vi "Sprinkler.vi"() -> ()   [LabVIEW 2024]
uses:
  Controls/Data Cluster.ctl
  <vilib>/Utility/error.llb/Error Cluster From Error Code.vi
  <vilib>/ErrorRing/Error Ring.xnode
panel:
  in  "Error In":errorcluster
  in  "Zone Setup Array":cluster{"Zone Selector":string, "Timing":dbl}[](array[cluster])
  out "Controller Status":string
  out "Zone Indicators":T1
  in  "Water Pressure Sensor (%)":u32(slide) scale=0.0..100.0
  in  "Rain Sensor":bool
  in  "Run Selector":bool
  in  "Setup":bool
  in  "Start":bool
  in  "stop":bool
  # "Controls"
  # "Simulation Controls"
  # "Rain"
  # "No Rain"
  # "Continuous"
  # "Single"
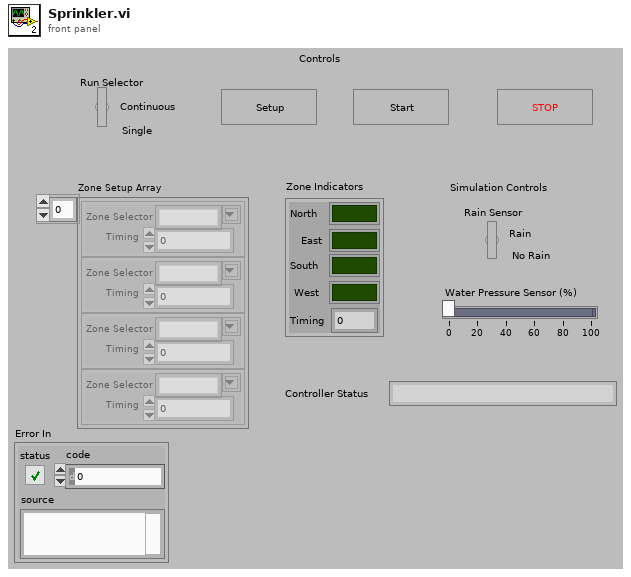
[diagram p1: front panel]
types:
  T1 = cluster{"North":bool, "East":bool, "South":bool, "West":bool, "Timing":u32}
  T2 = enum16{"Create", "Enqueue", "Dequeue", "Enstack", "Flush", "Release"}
  T3 = enum8{"Enabled", "Disabled", "Disabled and Grayed Out"}
  T4 = typedef "Data Cluster.ctl" = cluster{"Zone Setup Array Actual":cluster{"Zone Selector":string, "Timing":dbl}[], "Zone Setup Array Current":cluster{"Zone Selector":string, "Timing":dbl}[], "Zone Indicators":cluster{"North":bool, "East":bool, "South":bool, "West":bool, "Timing":u32}, "Controller Status":string, "Water Pressure Sensor (%)":u32, "Rain Sensor":bool, "Current Zone Active?":bool, "Time Elapsed?":bool, "QueueRefOut":refnum<queue>}
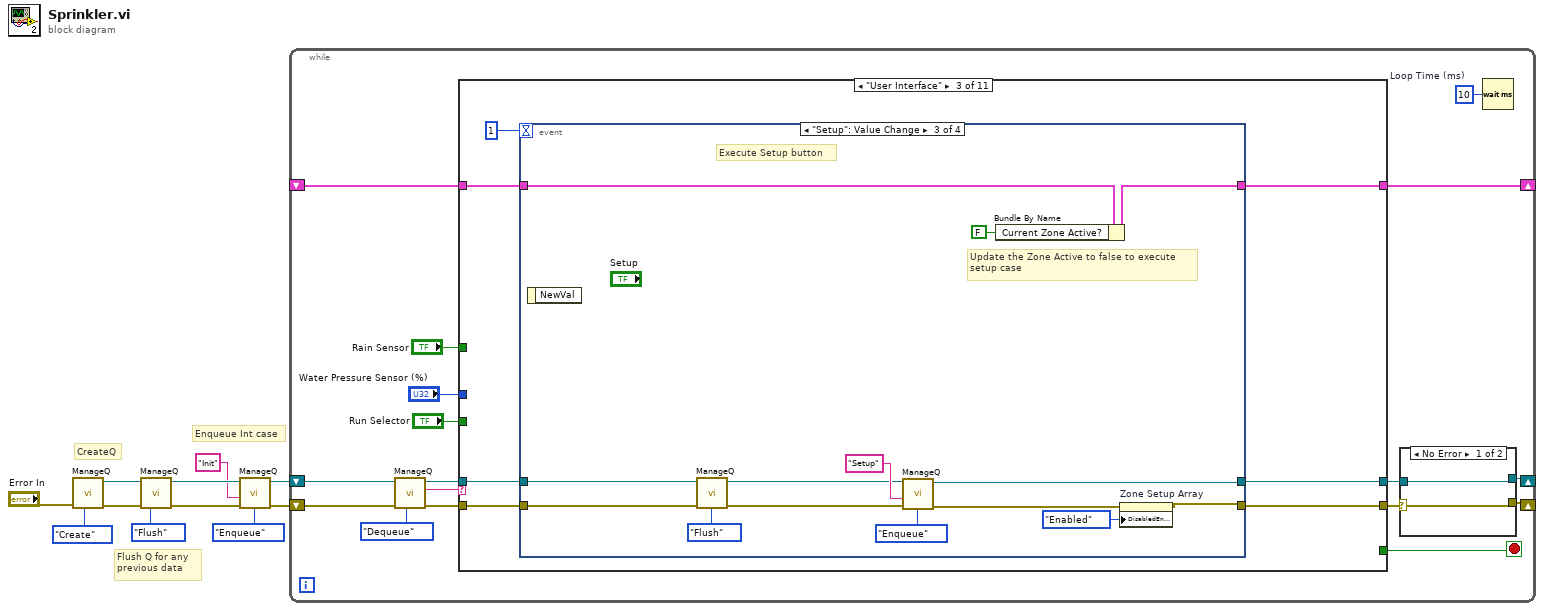
[diagram p0: block diagram]
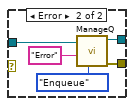
[diagram p2: hidden frame]
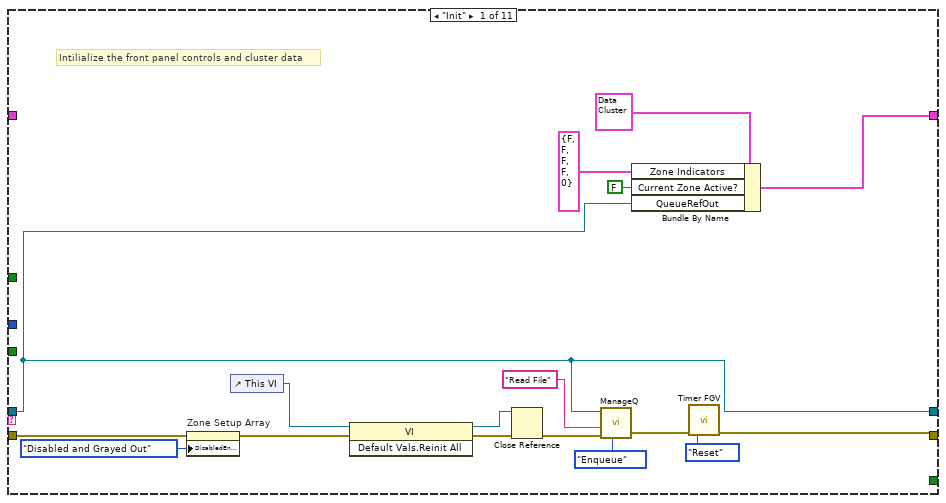
[diagram p3: hidden frame]
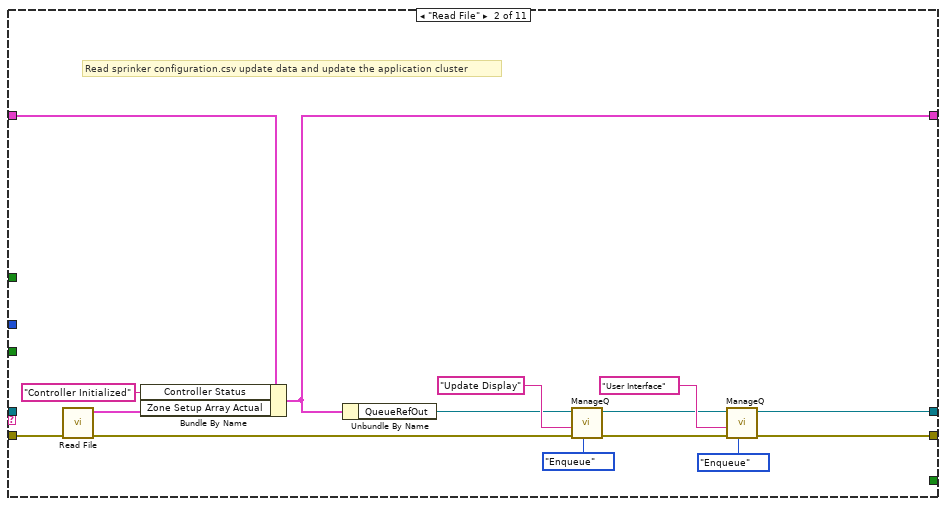
[diagram p4: hidden frame]
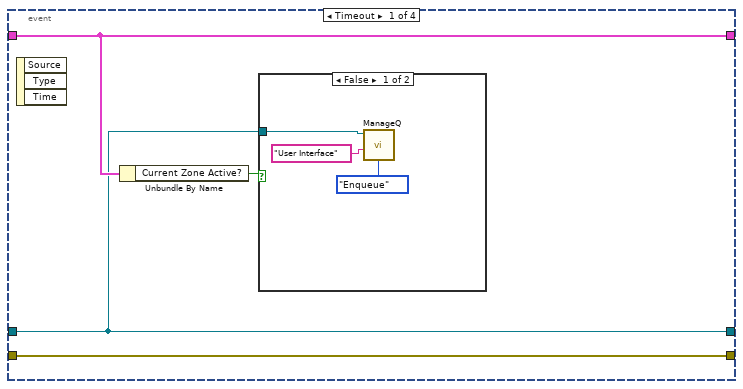
[diagram p5: hidden frame]
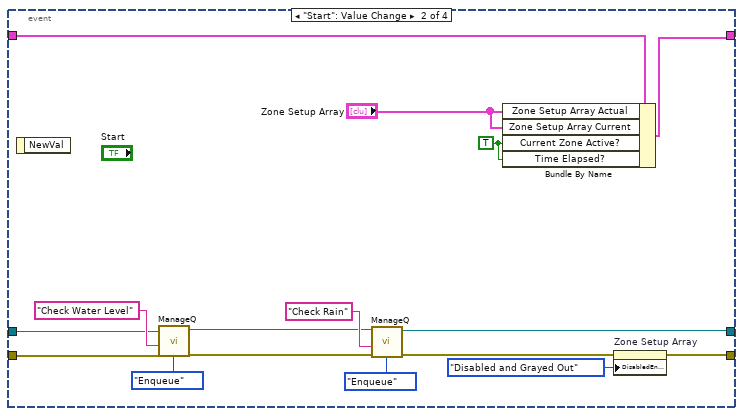
[diagram p7: hidden frame]
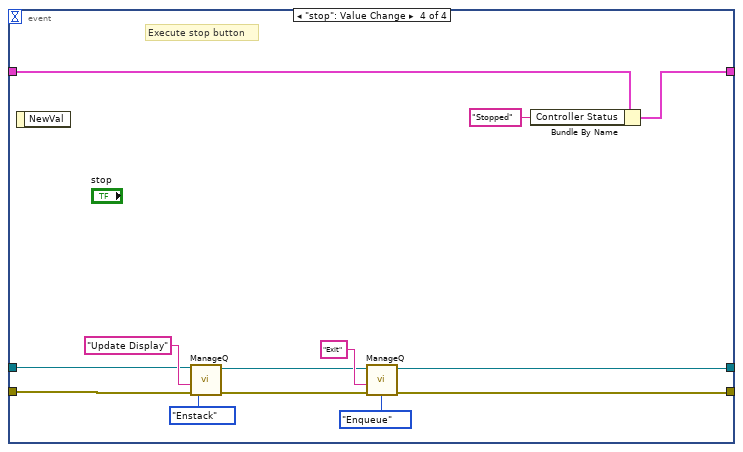
[diagram p8: hidden frame]
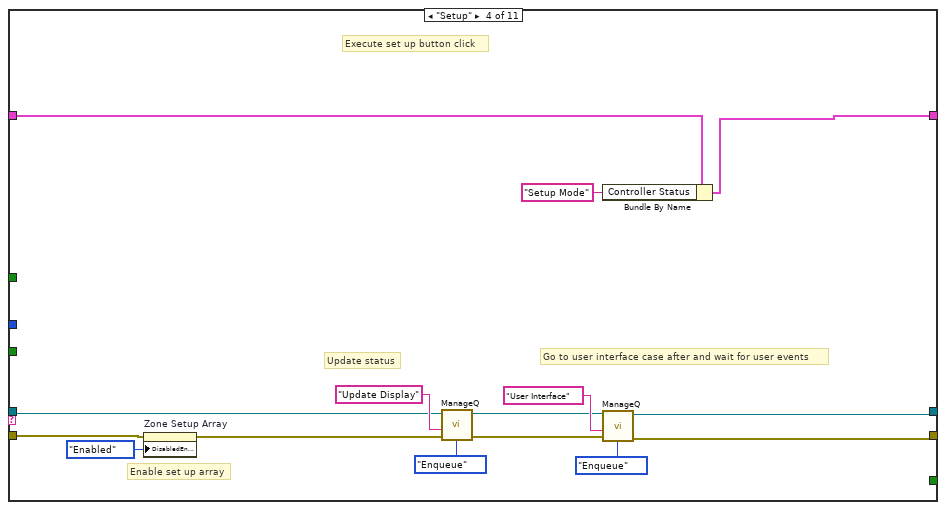
[diagram p9: hidden frame]
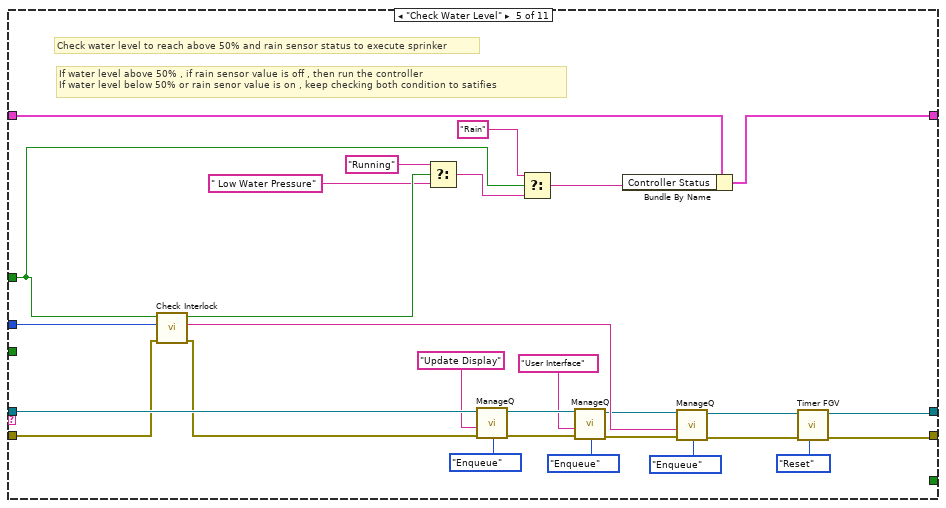
[diagram p10: hidden frame]
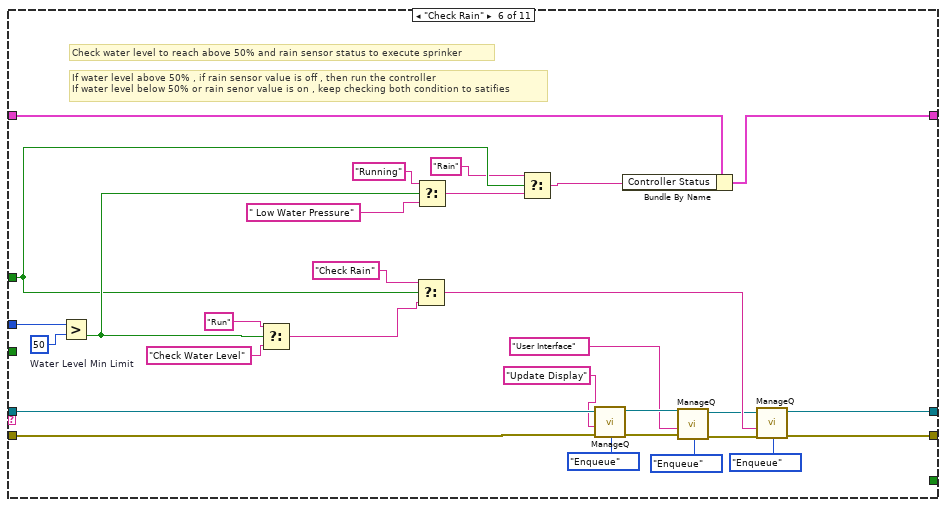
[diagram p11: hidden frame]
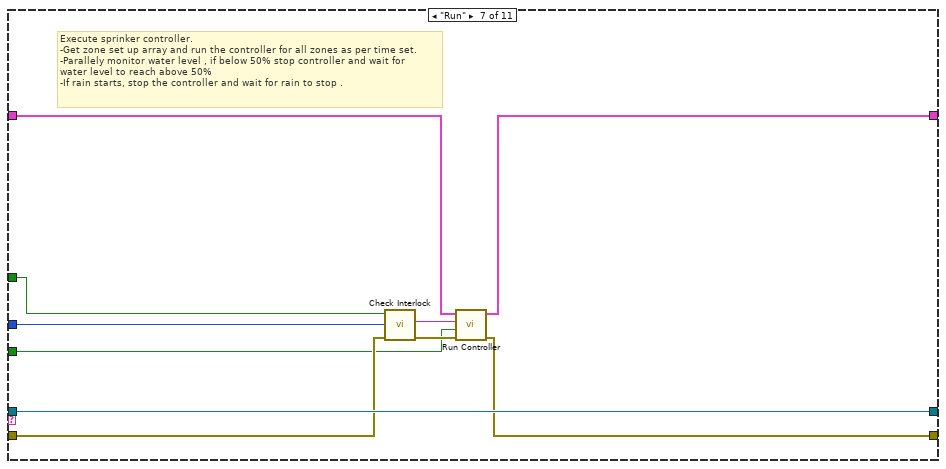
[diagram p12: hidden frame]
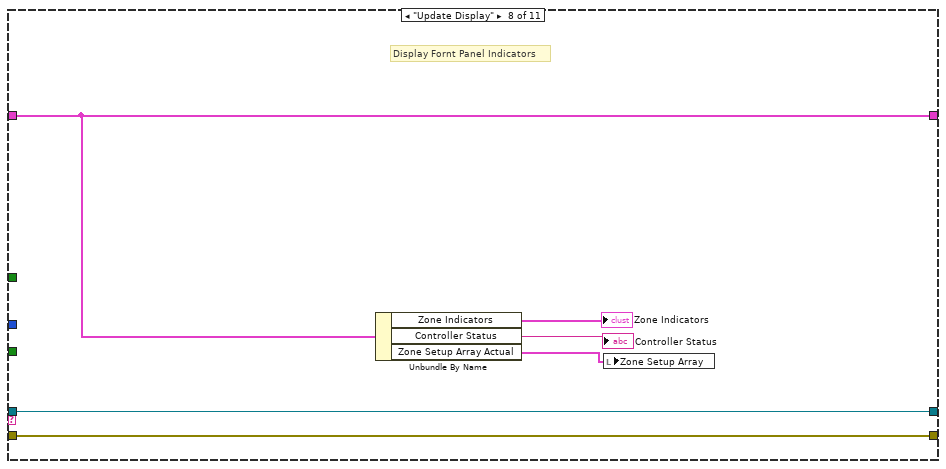
[diagram p13: hidden frame]
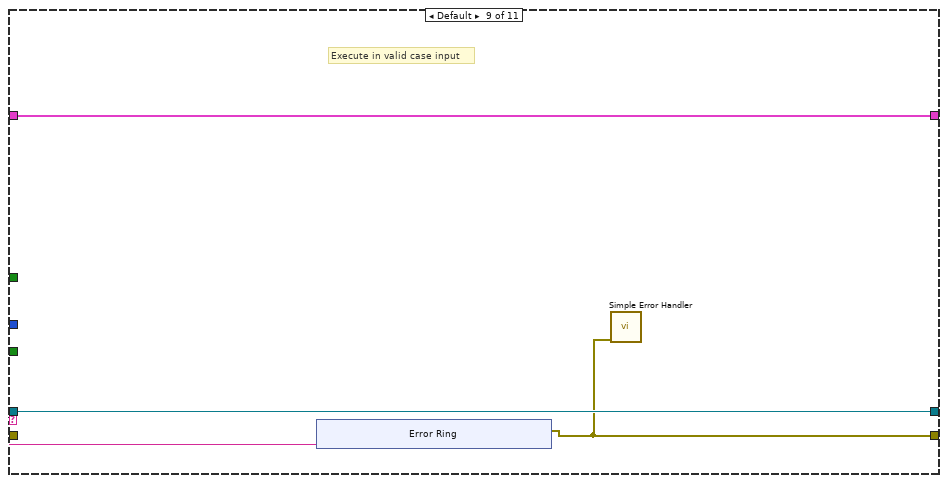
[diagram p14: hidden frame]
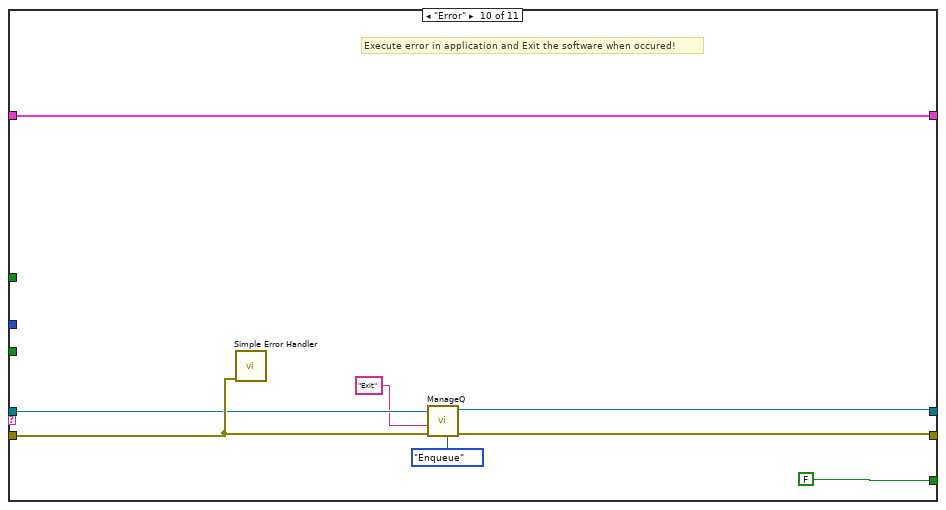
[diagram p15: hidden frame]
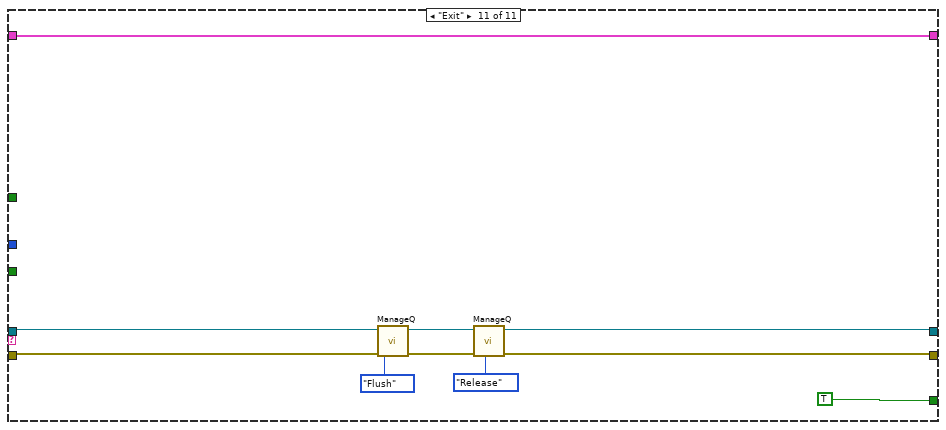
[diagram p16: hidden frame]
diagram:
  # "Enqueue Int case"
  # "Flush Q for any \nprevious data"
  # "CreateQ"
  n1 = call "ManageQ.vi"("QStateIn"=T2."Create", "Error In"="Error In") -> ("Error Out"=w9:errorcluster, "QueueRefOut"=w3:refnum<queue>)  [unwired: 7 in, 1 out]
  n2 = call "ManageQ.vi"("QStateIn"=T2."Flush", "Error In"=w9, "QueueRefIn"=w3) -> ("Error Out"=w8:errorcluster, "QueueRefOut"=w4:refnum<queue>)  [unwired: 6 in, 1 out]
  n3 = call "ManageQ.vi"("QStateIn"=T2."Enqueue", "Error In"=w8, "State In"="Init", "QueueRefIn"=w4) -> ("Error Out"=w7:errorcluster, "QueueRefOut"=w1:refnum<queue>)  [unwired: 5 in, 1 out]
  n4 = while {
    shift-right: [w19] -> _
    shift-left: w7 -> [w28]
    shift-right: [w21] -> _
    shift-left: _ -> [w22]
    shift-right: [w17] -> _
    shift-left: w1 -> [w26]
    stop <- w16 stop-if-true
    w15 = u32 10  # Loop Time (ms)
    n5 = call "ManageQ.vi"("QStateIn"=T2."Dequeue", "Error In"=w28, "QueueRefIn"=w26) -> ("Error Out"=w27:errorcluster, "State Out"=w24:string, "QueueRefOut"=w23:refnum<queue>)  [unwired: 6 in]
    n6 = case shown="\"User Interface\"" w24 {
      selector: w24 -> [_ _ _ _ _ _ _ _ w212 _ _]
      tunnel: w27 -> [w43 w67 w71 w138 w156 w192 w198 w210 _ w226 w236]
      tunnel: [w39 w55 w70 w133 w139 w191 w203 w210 w211 w223 w232] -> w20
      tunnel: w23 -> [w36 _ w72 w126 w164 w190 w204 w206 w213 w225 w237]
      tunnel: w22 -> [_ w66 w74 w131 w163 w186 w202 w209 w214 w229 w239]
      tunnel: [w45 w54 w73 w130 w157 w180 w201 w209 w214 w229 w239] -> w21
      tunnel: [w36 w58 w69 w134 w154 w189 w204 w206 w213 w224 w231] -> w18
      tunnel: [_ _ _ _ _ _ _ _ _ FALSE TRUE] -> w16
      tunnel: "Water Pressure Sensor (%)" -> [_ _ _ _ w165 w194 w199 _ _ _ _]
      tunnel: "Rain Sensor" -> [_ _ _ _ w159 w182 w200 _ _ _ _]
      tunnel: "Run Selector" -> [_ _ _ _ _ _ w195 _ _ _ _]
      frame "Init" {
        # "Intilialize the front panel controls and cluster data"
        n7 = property on="Zone Setup Array" class="Arr (strict)"(error in=w43, "DisabledEnum"=T3."Disabled and Grayed Out" ("Disabled")) -> (error out=w42:errorcluster)  [unwired: 1 in, 1 out]
        n8 = control-ref of="This VI"() -> (w52:refnum<vi>)
        n9 = invoke class="VI" method="Default Vals.Reinit All"(reference=w52, error in=w42) -> (reference out=w50:refnum<vi>, error out=w51:errorcluster)  [unwired: 1 in, 1 out]
        n10 = Close Reference(reference=w50, error in (no error)=w51) -> (error out=w49:errorcluster)
        n11 = call "ManageQ.vi"("QStateIn"=T2."Enqueue", "Error In"=w49, "State In"="Read File", "QueueRefIn"=w36) -> ("Error Out"=w40:errorcluster)  [unwired: 5 in, 2 out]
        n12 = Bundle By Name(cluster=T4 {"Zone Setup Array Actual"=[], "Zone Setup Array Current"=[], "Zone Indicators"={"North"=FALSE, "East"=FALSE, "South"=FALSE, "West"=FALSE, "Timing"=0}, "Controller Status"="", "Water Pressure Sensor (%)"=0, "Rain Sensor"=FALSE, "Current Zone Active?"=FALSE, "Time Elapsed?"=FALSE, "QueueRefOut"=refnum}, "Zone Indicators"=T1 {"North"=FALSE, "East"=FALSE, "South"=FALSE, "West"=FALSE, "Timing"=0}, "Current Zone Active?"=FALSE, "QueueRefOut"=w36) -> (w45:T4)
        n13 = call "Timer FGV.vi"("Error In"=w40, "Timer state"=enum16{"Reset", "Read", "Pause"}."Reset") -> ("Error Out"=w39:errorcluster)  [unwired: 7 in, 2 out]
      }
      frame "Read File" {
        # "Read sprinker configuration.csv update data and update the application cluster"
        n14 = call "Read File.vi"("Error In"=w67) -> ("Error Out"=w64:errorcluster, "Zone Set Up"=w65:cluster{"Zone Selector":string, "Timing":dbl}[])  [unwired: 9 in]
        n15 = Bundle By Name(cluster=w66, "Controller Status"="Controller Initialized", "Zone Setup Array Actual"=w65) -> (w54:T4)
        n16 = Unbundle By Name(w54) -> ("QueueRefOut"=w53:refnum<queue>)
        n17 = call "ManageQ.vi"("QStateIn"=T2."Enqueue", "Error In"=w64, "State In"="Update Display", "QueueRefIn"=w53) -> ("Error Out"=w56:errorcluster, "QueueRefOut"=w59:refnum<queue>)  [unwired: 5 in, 1 out]
        n18 = call "ManageQ.vi"("QStateIn"=T2."Enqueue", "Error In"=w56, "State In"="User Interface", "QueueRefIn"=w59) -> ("Error Out"=w55:errorcluster, "QueueRefOut"=w58:refnum<queue>)  [unwired: 5 in, 1 out]
      }
      frame "User Interface" {
        n19 = event shown="[2] \"Setup\": Value Change" {
          selector: _ -> [_ _ _ _]
          dyn-events: _ -> [_ _ _ _]
          timeout: 1 -> [_ _ _ _]
          tunnel: w74 -> [w77 w88 w103 w120]
          tunnel: [w77 w87 w102 w119] -> w73
          tunnel: w72 -> [w75 w92 w107 w115]
          tunnel: w71 -> [w78 w93 w106 w116]
          tunnel: [w78 w82 w98 w122] -> w70
          tunnel: [w75 w89 w109 w121] -> w69
          event Timeout {
            n20 = event-data() -> ()  [unwired: 1 in, 3 out]
            n21 = Unbundle By Name(w77) -> ("Current Zone Active?"=w76:bool)
            n22 = case shown="False" w76 {
              tunnel: w75 -> [w79 _]
              frame False {
                n23 = call "ManageQ.vi"("QStateIn"=T2."Enqueue", "State In"="User Interface", "QueueRefIn"=w79) -> ()  [unwired: 6 in, 3 out]
              }
              frame True {
              }
            }
          }
          event "Start": Value Change {
            w85 = TRUE ("Current Zone Active?")
            n24 = event-data() -> ()  [unwired: 1 in, 1 out]
            n25 = call "ManageQ.vi"("QStateIn"=T2."Enqueue", "Error In"=w93, "State In"="Check Water Level", "QueueRefIn"=w92) -> ("Error Out"=w90:errorcluster, "QueueRefOut"=w91:refnum<queue>)  [unwired: 5 in, 1 out]
            n26 = call "ManageQ.vi"("QStateIn"=T2."Enqueue", "Error In"=w90, "State In"="Check Rain", "QueueRefIn"=w91) -> ("Error Out"=w83:errorcluster, "QueueRefOut"=w89:refnum<queue>)  [unwired: 5 in, 1 out]
            n27 = Bundle By Name(cluster=w88, "Zone Setup Array Actual"="Zone Setup Array", "Zone Setup Array Current"="Zone Setup Array", "Current Zone Active?"=w85, "Time Elapsed?"=w85) -> (w87:T4)
            n28 = property on="Zone Setup Array" class="Arr (strict)"(error in=w83, "DisabledEnum"=T3."Disabled and Grayed Out" ("Disabled")) -> (error out=w82:errorcluster)  [unwired: 1 in, 1 out]
          }
          event "Setup": Value Change {
            # "Update the Zone Active to false to execute \nsetup case"
            # "Execute Setup button"
            n29 = event-data() -> ()  [unwired: 1 in, 1 out]
            n30 = call "ManageQ.vi"("QStateIn"=T2."Flush", "Error In"=w106, "QueueRefIn"=w107) -> ("Error Out"=w104:errorcluster, "QueueRefOut"=w105:refnum<queue>)  [unwired: 6 in, 1 out]
            n31 = call "ManageQ.vi"("QStateIn"=T2."Enqueue", "Error In"=w104, "State In"="Setup", "QueueRefIn"=w105) -> ("Error Out"=w99:errorcluster, "QueueRefOut"=w109:refnum<queue>)  [unwired: 5 in, 1 out]
            n32 = Bundle By Name(cluster=w103, "Current Zone Active?"=FALSE) -> (w102:T4)
            n33 = property on="Zone Setup Array" class="Arr (strict)"(error in=w99, "DisabledEnum"=T3."Enabled" ("Disabled")) -> (error out=w98:errorcluster)  [unwired: 1 in, 1 out]
          }
          event "stop": Value Change {
            # "Execute stop button"
            n34 = event-data() -> ()  [unwired: 1 in, 1 out]
            n35 = call "ManageQ.vi"("QStateIn"=T2."Enstack", "Error In"=w116, "State In"="Update Display", "QueueRefIn"=w115) -> ("Error Out"=w113:errorcluster, "QueueRefOut"=w114:refnum<queue>)  [unwired: 5 in, 1 out]
            n36 = call "ManageQ.vi"("QStateIn"=T2."Enqueue", "Error In"=w113, "State In"="Exit", "QueueRefIn"=w114) -> ("Error Out"=w122:errorcluster, "QueueRefOut"=w121:refnum<queue>)  [unwired: 5 in, 1 out]
            n37 = Bundle By Name(cluster=w120, "Controller Status"="Stopped") -> (w119:T4)
          }
        }
      }
      frame "Setup" {
        # "Update status"
        # "Go to user interface case after and wait for user events"
        # "Enable set up array"
        # "Execute set up button click"
        n38 = property on="Zone Setup Array" class="Arr (strict)"(error in=w138, "DisabledEnum"=T3."Enabled" ("Disabled")) -> (error out=w135:errorcluster)  [unwired: 1 in, 1 out]
        n39 = call "ManageQ.vi"("QStateIn"=T2."Enqueue", "State In"="Update Display", "QueueRefIn"=w126) -> ("QueueRefOut"=w125:refnum<queue>)  [unwired: 6 in, 2 out]
        n40 = Bundle By Name(cluster=w131, "Controller Status"="Setup Mode") -> (w130:T4)
        n41 = call "ManageQ.vi"("QStateIn"=T2."Enqueue", "Error In"=w135, "State In"="User Interface", "QueueRefIn"=w125) -> ("Error Out"=w133:errorcluster, "QueueRefOut"=w134:refnum<queue>)  [unwired: 5 in, 1 out]
      }
      frame "Check Water Level" {
        # "If water level above 50% , if rain sensor value is off , then run the controller\nIf water level below 50% or rain senor value is on , keep checking both condition to satifies"
        # "Check water level to reach above 50% and rain sensor status to execute sprinker"
        n42 = call "Check Interlock.vi"("Error In"=w156, "Water Pressure Sensor (%)"=w165, "Rain Sensor"=w159) -> ("Error Out"=w155:errorcluster, "State In"=w153:string, "Water Ok?"=w162:bool)  [unwired: 6 in]
        n43 = Select(t="Running" ("State In"), s=w162, f=" Low Water Pressure" ("State In")) -> (s? t:f=w142:string)
        n44 = call "ManageQ.vi"("QStateIn"=T2."Enqueue", "Error In"=w155, "State In"="Update Display", "QueueRefIn"=w164) -> ("Error Out"=w148:errorcluster, "QueueRefOut"=w149:refnum<queue>)  [unwired: 5 in, 1 out]
        n45 = Select(t="Rain" ("State In"), s=w159, f=w142) -> (s? t:f=w158:string)
        n46 = call "ManageQ.vi"("QStateIn"=T2."Enqueue", "Error In"=w148, "State In"="User Interface", "QueueRefIn"=w149) -> ("Error Out"=w144:errorcluster, "QueueRefOut"=w145:refnum<queue>)  [unwired: 5 in, 1 out]
        n47 = Bundle By Name(cluster=w163, "Controller Status"=w158) -> (w157:T4)
        n48 = call "ManageQ.vi"("QStateIn"=T2."Enqueue", "Error In"=w144, "State In"=w153, "QueueRefIn"=w145) -> ("Error Out"=w140:errorcluster, "QueueRefOut"=w154:refnum<queue>)  [unwired: 5 in, 1 out]
        n49 = call "Timer FGV.vi"("Error In"=w140, "Timer state"=enum16{"Reset", "Read", "Pause"}."Reset") -> ("Error Out"=w139:errorcluster)  [unwired: 7 in, 2 out]
      }
      frame "Check Rain" {
        w193 = u32 50  # Water Level Min Limit
        # "If water level above 50% , if rain sensor value is off , then run the controller\nIf water level below 50% or rain senor value is on , keep checking both condition to satifies"
        # "Check water level to reach above 50% and rain sensor status to execute sprinker"
        n50 = Greater?(x=w194, y=w193) -> (0:w185:bool)
        n51 = Select(t="Run" ("State In"), s=w185, f="Check Water Level" ("State In")) -> (s? t:f=w167:string)
        n52 = Select(t="Check Rain" ("State In"), s=w182, f=w167) -> (s? t:f=w179:string)
        n53 = Select(t="Running" ("State In"), s=w185, f=" Low Water Pressure" ("State In")) -> (s? t:f=w168:string)
        n54 = Select(t="Rain" ("State In"), s=w182, f=w168) -> (s? t:f=w181:string)
        n55 = call "ManageQ.vi"("QStateIn"=T2."Enqueue", "Error In"=w192, "State In"="Update Display", "QueueRefIn"=w190) -> ("Error Out"=w173:errorcluster, "QueueRefOut"=w175:refnum<queue>)  [unwired: 5 in, 1 out]
        n56 = Bundle By Name(cluster=w186, "Controller Status"=w181) -> (w180:T4)
        n57 = call "ManageQ.vi"("QStateIn"=T2."Enqueue", "Error In"=w173, "State In"="User Interface", "QueueRefIn"=w175) -> ("Error Out"=w172:errorcluster, "QueueRefOut"=w174:refnum<queue>)  [unwired: 5 in, 1 out]
        n58 = call "ManageQ.vi"("QStateIn"=T2."Enqueue", "Error In"=w172, "State In"=w179, "QueueRefIn"=w174) -> ("Error Out"=w191:errorcluster, "QueueRefOut"=w189:refnum<queue>)  [unwired: 5 in, 1 out]
      }
      frame "Run" {
        # "Execute sprinker controller.\n-Get zone set up array and run the controller for all zones as per time set.\n-Parallely monitor water level , if below 50% stop controller and wait for \nwater level to reach above 50%\n-If rain starts, stop the controller and wait for rain to stop ."
        n59 = call "Check Interlock.vi"("Error In"=w198, "Water Pressure Sensor (%)"=w199, "Rain Sensor"=w200) -> ("Error Out"=w197:errorcluster, "State In"=w196:string)  [unwired: 6 in, 1 out]
        n60 = call "Run Controller.vi"("Error In"=w197, "Run Selector"=w195, "Interlock Check Output"=w196, "Cluster Data In"=w202) -> ("Error Out"=w203:errorcluster, "Cluster Data Out"=w201:T4)  [unwired: 6 in]
      }
      frame "Update Display" {
        # "Display Fornt Panel Indicators"
        n61 = Unbundle By Name(w209) -> ("Zone Indicators"=→"Zone Indicators":T1, "Controller Status"=→"Controller Status":string, "Zone Setup Array Actual"=w205:cluster{"Zone Selector":string, "Timing":dbl}[])
        n62 = local write "Zone Setup Array"(w205) -> ()
      }
      frame Default {
        # "Execute in valid case input"
        n63 = xnode "Error Ring"("parameter 0"=w212) -> ("error out"=w211:errorcluster)
        n64 = call <vilib>:"Simple Error Handler.vi"("error in (no error)"=w211) -> ()  [unwired: 4 in, 5 out]
      }
      frame "Error" {
        # "Execute error in application and Exit the software when occured!"
        n65 = call <vilib>:"Simple Error Handler.vi"("error in (no error)"=w226) -> ()  [unwired: 4 in, 5 out]
        n66 = call "ManageQ.vi"("QStateIn"=T2."Enqueue", "Error In"=w226, "State In"="Exit", "QueueRefIn"=w225) -> ("Error Out"=w223:errorcluster, "QueueRefOut"=w224:refnum<queue>)  [unwired: 5 in, 1 out]
      }
      frame "Exit" {
        n67 = call "ManageQ.vi"("QStateIn"=T2."Flush", "Error In"=w236, "QueueRefIn"=w237) -> ("Error Out"=w235:errorcluster, "QueueRefOut"=w233:refnum<queue>)  [unwired: 6 in, 1 out]
        n68 = call "ManageQ.vi"("QStateIn"=T2."Release", "Error In"=w235, "QueueRefIn"=w233) -> ("Error Out"=w232:errorcluster, "QueueRefOut"=w231:refnum<queue>)  [unwired: 6 in, 1 out]
      }
    }
    n69 = case shown="No Error" w20 {
      selector: w20 -> [w29 _]
      tunnel: [w29 w35] -> w19
      tunnel: w18 -> [w30 w34]
      tunnel: [w30 w33] -> w17
      frame No Error {
      }
      frame Error {
        n70 = call "ManageQ.vi"("QStateIn"=T2."Enqueue", "State In"="Error", "QueueRefIn"=w34) -> ("Error Out"=w35:errorcluster, "QueueRefOut"=w33:refnum<queue>)  [unwired: 6 in, 1 out]
      }
    }
    n71 = Wait (ms)(milliseconds to wait=w15) -> ()  [unwired: 1 out]
  }
